vi "test_Object Tracking.vi"() -> ()   [LabVIEW 2020]
doc: "This example demonstrates the Traditional MeanShift algorithm to track an object in the image."
uses:
  <vilib>/vision/NI_Vision_Development_Module.lvlib
panel:
  in  "Stop":bool
  in  "Delay (s.)":dbl(slide) scale=0.0..2.0
  out "Image":T1(plugin-control)
  # "Overview: Demonstrate the Traditional MeanShift algorithm to track an object in the image.\nRequirements: LabVIEW Full Development System and Vision Development Module.\nInstructions: Run the VI."
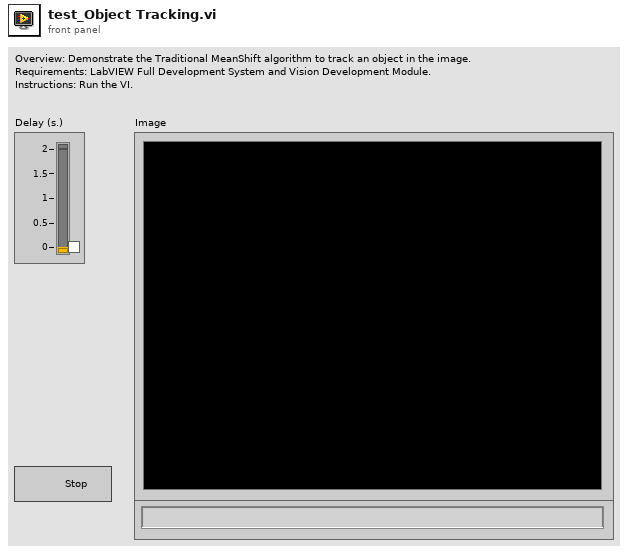
[diagram p1: front panel]
types:
  T1 = typedef "IMAQ Image.ctl" = refnum<image>
  T2 = typedef "Image Type" = u32
  T3 = cluster{"Number of Histogram Bins":i32, "Blending Parameter (%)":dbl, "Maximum Iterations":i32}
  T4 = typedef "IMAQ Object Tracking Session.ctl" = refnum<k20>
  T5 = typedef "IMAQ Rectangle" = cluster{"Left":i32, "Top":i32, "Right":i32, "Bottom":i32, "Rotation":dbl}
  T6 = typedef "ROI Descriptor" = cluster{"Global Rectangle":i32[], "Contours":cluster{"ID":enum32{"External", "Internal"}, "Type":u32, "Coordinates":i32[]}[]}
  T7 = cluster{"Label":string, "Score":i32, "Angle":dbl, "Location":cluster{"X":dbl, "Y":dbl}, "Bounding Box":cluster{"X":dbl, "Y":dbl}[], "Object Found?":bool}[]
  T8 = cluster{"Label":string, "Score":i32, "Angle":dbl, "Location":cluster{"X":dbl, "Y":dbl}, "Bounding Box":cluster{"X":dbl, "Y":dbl}[], "Object Found?":bool}
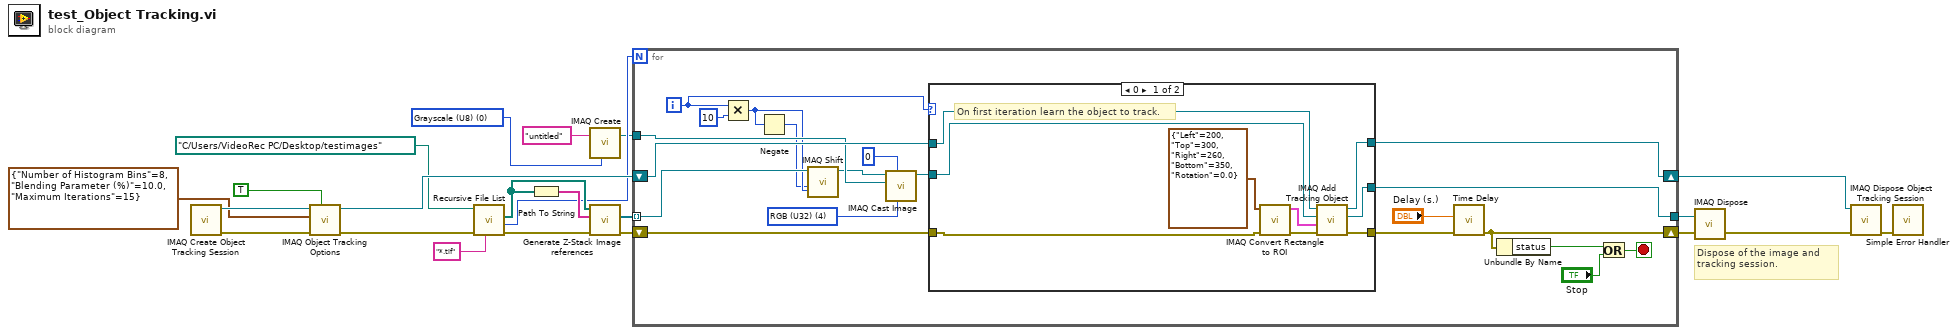
[diagram p0: block diagram]
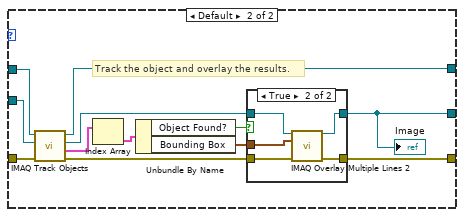
[diagram p2: hidden frame]
diagram:
  w2 = T2 0 items=["Grayscale (U8)", "Grayscale (I16)", "Grayscale (SGL)", "Complex (CSG)", "RGB (U32)", "HSL (U32)", "RGB (U64)", "Grayscale (U16)"] ("Image Type")
  # "Dispose of the image and tracking session."
  n1 = call "IMAQ Create Object Tracking Session"() -> ("error out"=w15:errorcluster, "Object Tracking Session"=w18:T4)  [unwired: 1 in, 9 out]
  n2 = call-poly "IMAQ Object Tracking Options"("Get/Set (Get)"=TRUE, "error in (no error)"=w15, "Mean Shift Options in"=T3 {"Number of Histogram Bins"=8, "Blending Parameter (%)"=10.0, "Maximum Iterations"=15}, "Object Tracking Session In"=w18) -> ("error out"=w5:errorcluster, "Object Tracking Session Out"=w17:T4)  [unwired: 5 in, 1 out]
  n3 = call <vilib>:"Recursive File List.vi"("pattern"="*.tif", "error in (no error)"=w5, "Folder Path"=path "C:/Users/VideoRec PC/Desktop/testimages" ("Experiment folder path OR Z-stack folder path")) -> ("error out"=w4:errorcluster, "Number of Files"=w7:i32, "All Files in Dir"=w10:path[])  [unwired: 4 in, 2 out]
  n4 = Path To String(path=w10) -> (string=w9:string[])
  n5 = call "IMAQ Create"("Image Name"="untitled", "Image Type"=w2) -> ("New Image"=w3:T1)  [unwired: 3 in, 1 out]
  n6 = call "Generate Z-Stack Image references.vi"("error in (no error)"=w4, "Channel File Names"=w9, "Channel File Paths"=w10) -> ("error out"=w6:errorcluster, "Image Array refs"=w8:T1[])  [unwired: 6 in, 1 out]
  n7 = for {
    N: w7 -> [_]
    tunnel: [w41] -> w22
    shift-right: [w39] -> w21
    shift-left: w17 -> [w40]
    shift-right: [w34] -> w13
    shift-left: w6 -> [w33]
    tunnel: w8 -> [w29] mode=indexing
    tunnel: w3 -> [w28]
    i -> [w25]
    stop <- w35 stop-if-true
    w31 = T2 4 items=["Grayscale (U8)", "Grayscale (I16)", "Grayscale (SGL)", "Complex (CSG)", "RGB (U32)", "HSL (U32)", "RGB (U64)", "Grayscale (U16)"] ("Image Type")
    n8 = Multiply(x=w25, y=10 ("Y Offset")) -> (x*y=w24:i32)
    n9 = Negate(x=w24) -> (-x=w23:i32)
    n10 = call "IMAQ Shift"("YOffset"=w24, "XOffset"=w23, "Image Src"=w29) -> ("Image Dst Out"=w27:T1)  [unwired: 7 in, 1 out]
    n11 = call "IMAQ Cast Image"("Image Type"=w31, "# Shifts"=0, "Image Dst"=w28, "Image Src"=w27) -> ("Image Dst Out"=w32:T1)  [unwired: 6 in, 1 out]
    n12 = case shown="0" w25 {
      tunnel: [w48 w63] -> w39
      tunnel: [w50 w60] -> w41
      tunnel: [w49 w56] -> w37
      tunnel: w40 -> [w51 w58]
      tunnel: w32 -> [w47 w54]
      tunnel: w33 -> [w46 w53]
      frame 0 {
        # "On first iteration learn the object to track."
        n13 = call "IMAQ Convert Rectangle to ROI"("error in (no error)"=w46, "Rectangle"=T5 {"Left"=200, "Top"=300, "Right"=260, "Bottom"=350, "Rotation"=0.0}) -> ("error out"=w45:errorcluster, "ROI Descriptor"=w44:T6)  [unwired: 7 in]
        n14 = call "IMAQ Add Tracking Object"("error in (no error)"=w45, "ROI Descriptor"=w44, "Image"=w47, "Object Tracking Session In"=w51) -> ("error out"=w49:errorcluster, "Image (duplicate)"=w50:T1, "Object Tracking Session Out"=w48:T4)  [unwired: 1 in, 4 out]
      }
      frame Default {
        # "Track the object and overlay the results."
        n15 = call "IMAQ Track Objects"("error in (no error)"=w53, "Image"=w54, "Object Tracking Session In"=w58) -> ("error out"=w57:errorcluster, "Objects (pixel)"=w62:T7, "Image (duplicate)"=w61:T1, "Object Tracking Session Out"=w63:T4)  [unwired: 1 in, 4 out]
        n16 = Index Array(array=w62) -> (element=w55:T8)  [unwired: 1 in]
        n17 = Unbundle By Name(w55) -> ("Object Found?"=w52:bool, "Bounding Box"=w59:cluster{"X":dbl, "Y":dbl}[])
        n18 = case shown="True" w52 {
          tunnel: w61 -> [w64 w70]
          tunnel: [w64 w69] -> w60
          tunnel: w59 -> [_ w68]
          tunnel: w57 -> [w65 w67]
          tunnel: [w65 w66] -> w56
          frame False {
          }
          frame True {
            n19 = call "IMAQ Overlay Multiple Lines 2"("Image"=w70, "Line End Points"=w68, "error in (no error)"=w67) -> ("Image Out"=w69:T1, "error out"=w66:errorcluster)  [unwired: 5 in, 6 out]
          }
        }
        "Image" <- w60
      }
    }
    n20 = call "Time Delay"("error in (no error)"=w37, "Delay Time (s)"="Delay (s.)") -> ("error out"=w34:errorcluster)  [unwired: 9 in]
    n21 = Unbundle By Name(w34) -> ("status"=w42:bool)
    n22 = Or(x=w42, y="Stop") -> (x .or. y?=w35:bool)
  }
  n23 = call "IMAQ Dispose"("Image"=w22, "error in (no error)"=w13) -> ("error out"=w20:errorcluster)  [unwired: 1 in, 3 out]
  n24 = call "IMAQ Dispose Object Tracking Session"("error in (no error)"=w20, "Object Tracking Session"=w21) -> ("error out"=w19:errorcluster)  [unwired: 9 out]
  n25 = call <vilib>:"Simple Error Handler.vi"("error in (no error)"=w19) -> ()  [unwired: 1 in, 8 out]
